vi "Voltage Nominal Write Single.vi"(8 "error in":errorcluster, 9 "Channel Index":i32=1, 10 "Voltage Nominal AV":dbl, 11 "Cycler in":refnum<class "Cycler.lvclass">) -> (0 "error out":errorcluster, 3 "Cycler out":refnum<class "Cycler.lvclass">)   [LabVIEW 2023, in "Cycler.lvclass"]
uses:
  Cycler.lvclass
  Low Level Capabilities/Voltage/Voltage Nominal Value/Voltage Nominal Value.lvclass
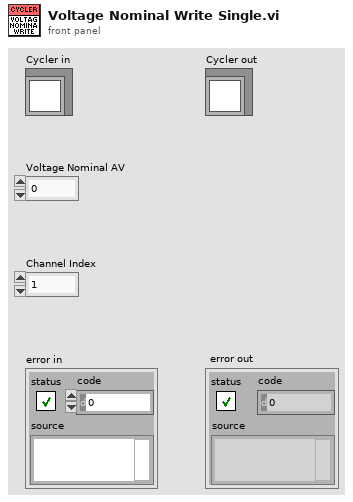
[diagram p1: front panel]
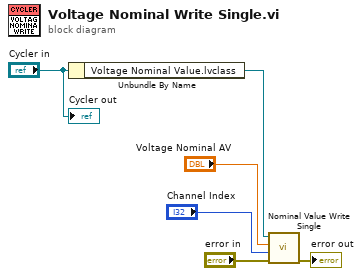
[diagram p0: block diagram]
diagram:
  n1 = Unbundle By Name("Cycler in") -> ("Voltage Nominal Value.lvclass"=w1:refnum<class "Voltage Nominal Value.lvclass">)
  n2 = call-dynamic "Nominal Value Write Single.vi"("error in"="error in", "Channel Index"="Channel Index", "Voltage Nominal Value"="Voltage Nominal AV", "Voltage Nominal Value in"=w1) -> ("error out"=→"error out":errorcluster)  [unwired: 6 in, 1 out]
  "Cycler out" <- "Cycler in"
